vi "Get Band 3 Value.vi"(11 "Color Band 3":T1 items=["Black"=0, "Brown"=1, "Red"=2, "Orange"=3, "Yellow"=4, "Green"=5, "Blue"=6, "Violet"=7, "Grey"=8, "White"=9, "Please Select"=11]) -> (3 "Multiplier":i32)   [LabVIEW 2012]
uses:
  Colors.ctl
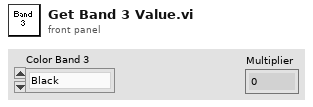
[diagram p1: front panel]
types:
  T1 = typedef "Colors.ctl" = u16
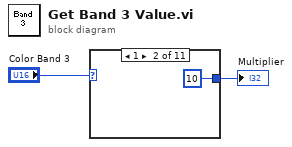
[diagram p0: block diagram]
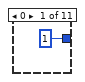
[diagram p2: hidden frame]
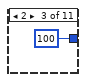
[diagram p3: hidden frame]
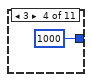
[diagram p4: hidden frame]
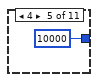
[diagram p5: hidden frame]
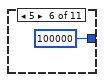
[diagram p6: hidden frame]
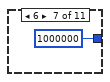
[diagram p7: hidden frame]
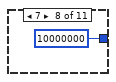
[diagram p8: hidden frame]
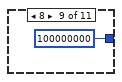
[diagram p9: hidden frame]
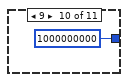
[diagram p10: hidden frame]
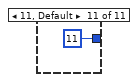
[diagram p11: hidden frame]
diagram:
  n1 = case shown="1" "Color Band 3" {
    tunnel: [1 10 100 1000 10000 100000 1000000 10000000 100000000 1000000000 11] -> w2
    frame 0 {
    }
    frame 1 {
    }
    frame 2 {
    }
    frame 3 {
    }
    frame 4 {
    }
    frame 5 {
    }
    frame 6 {
    }
    frame 7 {
    }
    frame 8 {
    }
    frame 9 {
    }
    frame 11, Default {
    }
  }
  "Multiplier" <- w2
